vi "connect PG server.vi"(8 "error in (no error)":errorcluster, 11 "SP in":refnum<class "PG analogs.lvclass">) -> (0 "error out":errorcluster, 2 "conn_out":u64, 3 "SP out":refnum<class "PG analogs.lvclass">)   [LabVIEW 2019, in "PG analogs.lvclass"]
uses:
  PG analogs.lvclass
  D:/my_projects/projects/Algorithms/Labview/19/Database/Save messages PGserver/Save messages PGserver.lvclass
  Save messages PGserver/Save messages PGserver.lvclass/Save messages PGserver.ctl
  PostgreSQL2LabVIEW/libpqlv/src/PQfinish.vi
  PostgreSQL2LabVIEW/libpqUtility/src/PQlistColumns.vi
  PostgreSQL2LabVIEW/libpqUtility/src/PQexecute.vi
  PostgreSQL2LabVIEW/libpqlv/src/PQconnectdb.vi
  PostgreSQL2LabVIEW/libpqlv/src/PQerrorMessage.vi
  PostgreSQL2LabVIEW/libpqlv/src/PQstatus.vi
  <vilib>/dlg_ctls.llb/Space Constant.vi
  PostgreSQL2LabVIEW/libpqUtility/src/PQgetColumn.vi
  PostgreSQL2LabVIEW/libpqlv/src/PQresultErrorMessage.vi
  PostgreSQL2LabVIEW/libpqUtility/src/PQclear.vi
  PostgreSQL2LabVIEW/libpqlv/src/PQsendQuery.vi
  PostgreSQL2LabVIEW/libpqlv/src/PQgetResult.vi
  PostgreSQL2LabVIEW/libpqlv/src/PQresultStatus.vi
  PostgreSQL2LabVIEW/libpqlv/src/PQclear.vi
  PostgreSQL2LabVIEW/libpqUtility/src/PQfetchTables.vi
  PostgreSQL2LabVIEW/libpqlv/src/PQgetvalue.vi
  PostgreSQL2LabVIEW/libpqlv/src/PQntuples.vi
  PostgreSQL2LabVIEW/libpqUtility64/libpqutility64.lvlib
  PostgreSQL.lvlib
  Save messages PGserver/Save messages PGserver.lvclass
  PostgreSQL2LabVIEW/libpqUtility/libpqutility.lvlib
panel:
  out "PQStatus":T1(ring)
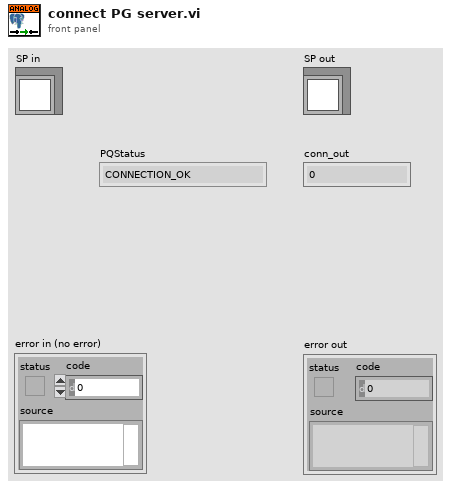
[diagram p1: front panel]
types:
  T1 = enum32{"CONNECTION_OK", "CONNECTION_BAD", "CONNECTION_STARTED", "CONNECTION_MADE", "CONNECTION_AWAITING_RESPONSE", "CONNECTION_AUTH_OK", "CONNECTION_SETENV", "CONNECTION_SSL_STARTUP", "CONNECTION_NEEDED"}
  T2 = typedef "PostgreSQL.lvlib/Coninfo.ctl" = cluster{"host":string, "port":string, "client_encoding":string, "dbname":string, "user":string, "password":string}
  T3 = typedef "Save messages PGserver.lvclass/table parameters.ctl" = cluster{"table postfix":string, "sequence name":string, "columns name":string[], "columns type":string}
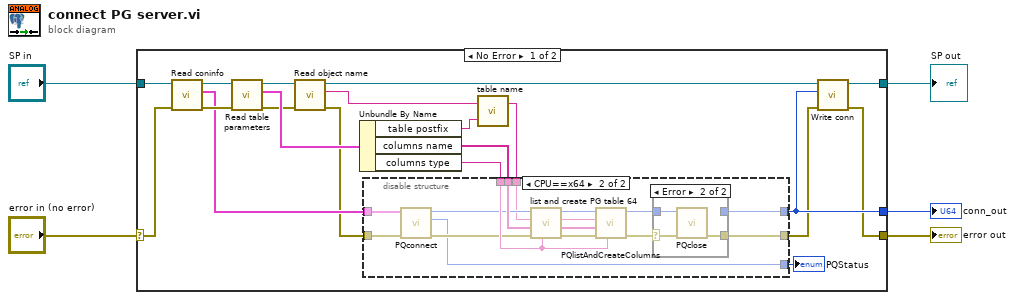
[diagram p0: block diagram]
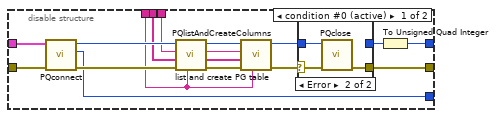
[diagram p2: hidden frame]
diagram:
  n1 = case shown="No Error" "error in (no error)" {
    selector: "error in (no error)" -> [w16 w65]
    tunnel: [w18 w65] -> w2
    tunnel: [w21 w66] -> w4
    tunnel: "SP in" -> [w17 w66]
    tunnel: [w20 _] -> w1
    frame No Error {
      n2 = call "Read coninfo.vi"("error in (no error)"=w16, "SP in"=w17) -> ("error out"=w14:errorcluster, "conninfo"=w13:T2, "SP out"=w15:refnum<class "PG analogs.lvclass">)  [unwired: 7 in]
      n3 = call "Read table parameters.vi"("error in (no error)"=w14, "SP in"=w15) -> ("error out"=w11:errorcluster, "table parameters"=w25:T3, "SP out"=w12:refnum<class "PG analogs.lvclass">)  [unwired: 7 in]
      n4 = call "Read object name.vi"("error in (no error)"=w11, "SP in"=w12) -> ("error out"=w10:errorcluster, "object name"=w9:string, "SP out"=w8:refnum<class "PG analogs.lvclass">)  [unwired: 7 in]
      n5 = Unbundle By Name(w25) -> ("table postfix"=w24:string, "columns name"=w23:string[], "columns type"=w22:string)
      n6 = call "table name.vi"("postfix"=w24, "object name"=w9) -> ("table name"=w7:string)  [unwired: 1 in]
      n7 = disable-structure shown="CPU==x64" {
        disable-tunnel: w7 -> [w26 w46]
        disable-tunnel: w23 -> [w27 w59]
        disable-tunnel: w22 -> [w29 w58]
        disable-tunnel: [w28 w57] -> w20
        disable-tunnel: [w39 w56] -> w19
        disable-tunnel: w13 -> [w38 w55]
        disable-tunnel: w10 -> [w37 w54]
        disable-tunnel: [w30 w47] -> w6
        frame condition #0 (active) {
          n8 = call "PQconnect.vi"("error in (no error)"=w37, "conninfo"=w38) -> ("error out"=w35:errorcluster, "PQStatus"=w30:T1, "conn"=w36:u32)  [unwired: 7 in]
          n9 = call "list and create PG table.vi"("columns type (real)"=w29, "error in"=w35, "columns"=w27, "table name"=w26, "conn"=w36) -> ("error out"=w32:errorcluster, "conn_out"=w34:u32)  [unwired: 5 in]
          n10 = call "PQlistAndCreateColumns.vi"("column type"=w29, "error in"=w32, "table"=w27, "table name"=w26, "conn"=w34) -> ("error out"=w31:errorcluster, "conn_out"=w33:u32)  [unwired: 5 in]
          n11 = case shown="Error" w31 {
            selector: w31 -> [w41 w44]
            tunnel: w33 -> [w42 w45]
            tunnel: [w42 _] -> w40
            tunnel: [w41 w43] -> w39
            frame No Error {
            }
            frame Error {
              n12 = call "PQclose.vi"("error in (no error)"=w44, "conn"=w45) -> ("error out"=w43:errorcluster)  [unwired: 9 in]
            }
          }
          n13 = To Unsigned Quad Integer(1:w40) -> (0:w28:u64)
        }
        frame condition #1 {
          n14 = call "PQconnect.vi"("error in (no error)"=w54, "conninfo"=w55) -> ("error out"=w52:errorcluster, "PQStatus"=w47:T1, "conn"=w53:u64)  [unwired: 7 in]
          n15 = call "list and create PG table 64.vi"("columns type (real)"=w58, "error in"=w52, "columns"=w59, "table name"=w46, "conn"=w53) -> ("error out"=w49:errorcluster, "conn_out"=w51:u64)  [unwired: 5 in]
          n16 = call "PQlistAndCreateColumns.vi"("column type"=w58, "error in"=w49, "table"=w59, "table name"=w46, "conn"=w51) -> ("error out"=w48:errorcluster, "conn_out"=w50:u64)  [unwired: 5 in]
          n17 = case shown="Error" w48 {
            selector: w48 -> [w60 w63]
            tunnel: w50 -> [w61 w64]
            tunnel: [w61 _] -> w57
            tunnel: [w60 w62] -> w56
            frame No Error {
            }
            frame Error {
              n18 = call "PQclose.vi"("error in (no error)"=w63, "conn"=w64) -> ("error out"=w62:errorcluster)  [unwired: 9 in]
            }
          }
        }
      }
      "PQStatus" <- w6
      n19 = call "Write conn.vi"("error in (no error)"=w19, "conn"=w20, "SP in"=w8) -> ("error out"=w18:errorcluster, "SP out"=w21:refnum<class "PG analogs.lvclass">)  [unwired: 7 in]
    }
    frame Error {
    }
  }
  "error out" <- w2
  "SP out" <- w4
  "conn_out" <- w1
